vi "ALARM (SubVI).vi"() -> ()   [LabVIEW 2017]
panel:
  out "INDICATOR":T1
  in  "SECURITY":T2
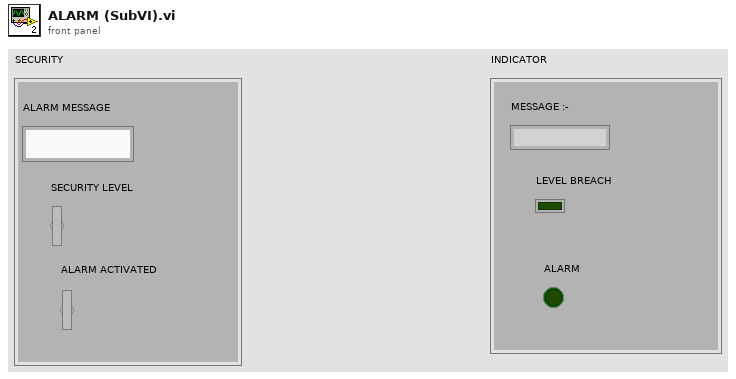
[diagram p1: front panel]
types:
  T1 = cluster{"MESSAGE :-":string, "LEVEL BREACH":bool, "ALARM":bool}
  T2 = cluster{"ALARM MESSAGE":string, "SECURITY LEVEL":bool, "ALARM ACTIVATED":bool}
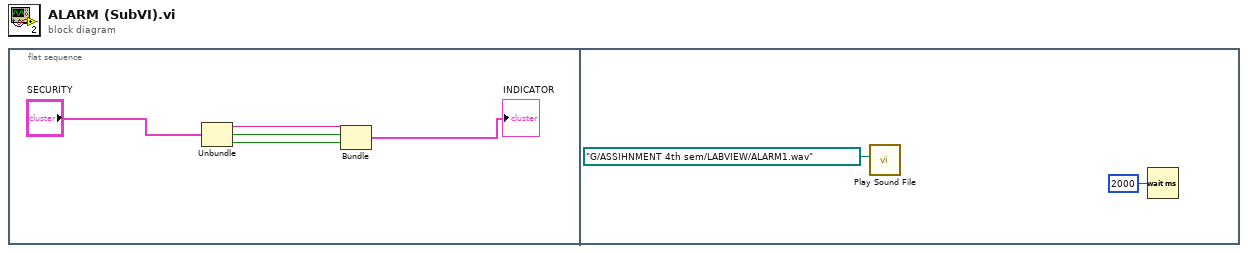
[diagram p0: block diagram]
diagram:
  n1 = flat-sequence {
    frame #0 {
      n2 = Unbundle("SECURITY") -> ("ALARM MESSAGE"=w4:string, "SECURITY LEVEL"=w3:bool, "ALARM ACTIVATED"=w2:bool)
      n3 = Bundle("ALARM MESSAGE"=w4, "SECURITY LEVEL"=w3, "ALARM ACTIVATED"=w2) -> (→"INDICATOR":T2)  [unwired: 1 in]
    }
    frame #1 {
      n4 = call <vilib>:"Play Sound File.vi"("path"=path "G:/ASSIHNMENT 4th sem/LABVIEW/ALARM1.wav") -> ()  [unwired: 9 in, 2 out]
      n5 = Wait (ms)(milliseconds to wait=u32 2000) -> ()  [unwired: 1 out]
    }
  }
